vi "CreateOutputPath.vi"(8 "error in (no error)":errorcluster, 11 "File to convert":path) -> (0 "error out":errorcluster, 3 "appended path":path)   [LabVIEW 2017]
uses:
  PathConfiguration.vi
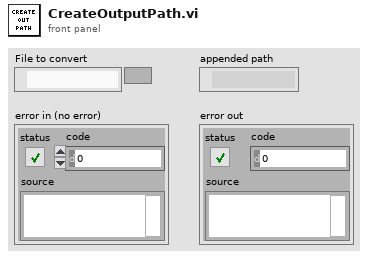
[diagram p1: front panel]
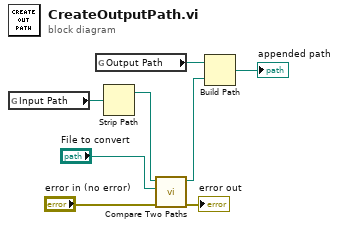
[diagram p0: block diagram]
diagram:
  n1 = global read "PathConfiguration.vi" "Input Path"() -> (w3:path)
  n2 = global read "PathConfiguration.vi" "Output Path"() -> (w1:path)
  n3 = Strip Path(path=w3) -> (stripped path=w4:path)  [unwired: 1 out]
  n4 = call <vilib>:"Compare Two Paths.vi"("error in (no error)"="error in (no error)", "Path 2"="File to convert", "Path 1"=w4) -> ("error out"=→"error out":errorcluster, "Relative Path from 1 to 2"=w6:path)  [unwired: 5 in, 2 out]
  n5 = Build Path(base path=w1, name or relative path=w6) -> (appended path=→"appended path":path)
